vi "6240AData_execute.vi"(0 "6240AData in":refnum<class "6240AData.lvclass">, 5 "SetCurrent (A)":dbl[](array[numeric]), 7 "FileFormat":string, 9 "Output status":bool[](array[boolean]), 10 "ExecutionIndex":i32, 11 "error in (no error)":errorcluster) -> (1 "ActualVoltage (V)":dbl[](array[numeric]), 3 "ActualCurrent (A)":dbl[](array[numeric]), 4 "6240AData out":refnum<class "6240AData.lvclass">, 6 "appended array":timestamp[](array[timestamp]), 12 "SetCurrentArray":dbl[][](array[numeric]), 14 "ActualCurrentArray":dbl[][](array[numeric]), 15 "error out":errorcluster)   [LabVIEW 2020, in "6240AData.lvclass"]
uses:
  6240AData.lvclass
  6240AData.lvclass/6240AData.ctl
  istr.lib/ADCMT 6240/Public/Configure/Configure Output Mode (DC).vi
  istr.lib/ADCMT 6240/Public/Action-Status/Output (Suspend).vi
  istr.lib/ADCMT 6240/Public/Action-Status/Output (Operate).vi
  istr.lib/ADCMT 6240/ADCMT 6240.lvlib
panel:
  out "appended array 2":dbl[](array[numeric])
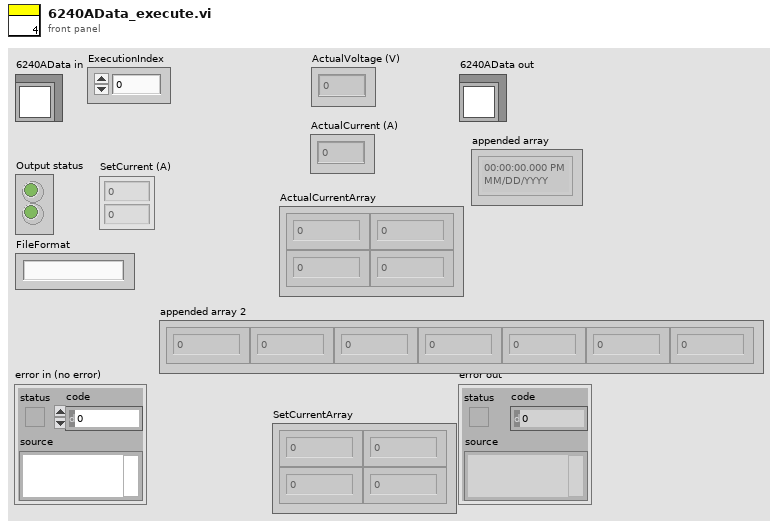
[diagram p1: front panel]
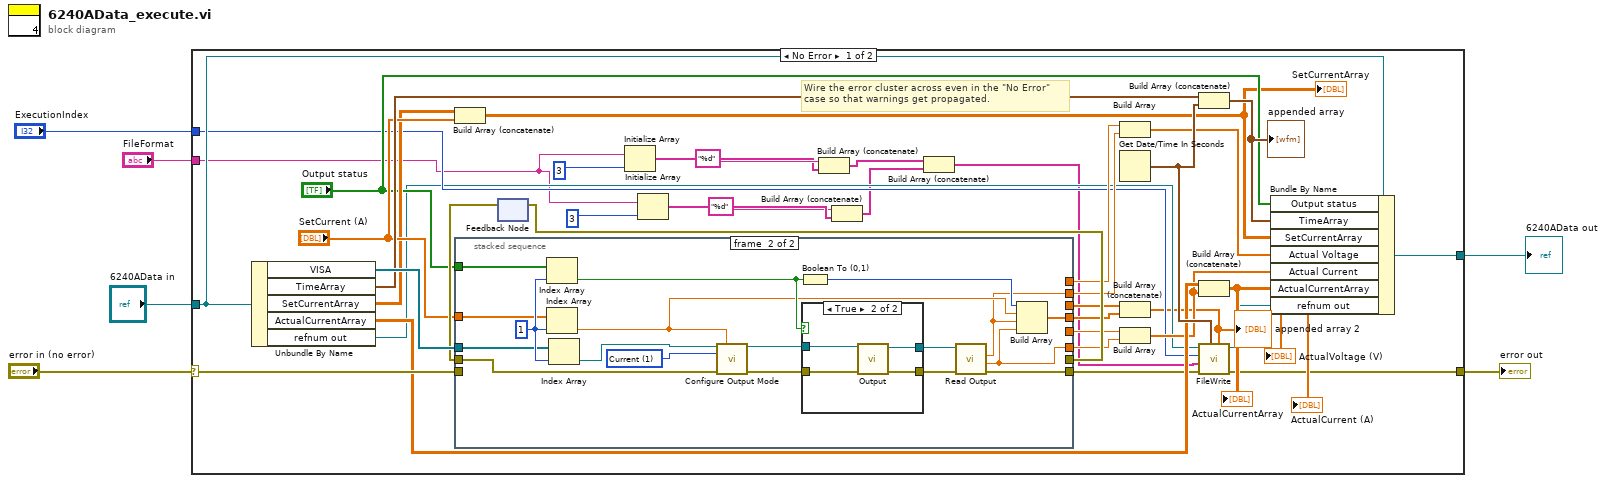
[diagram p0: block diagram]
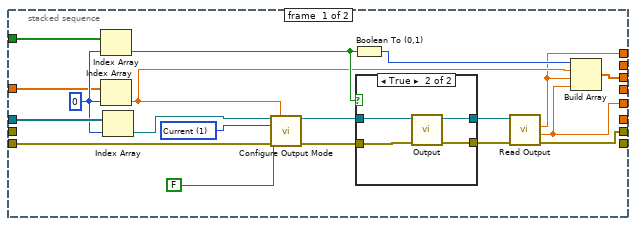
[diagram p2: hidden frame]
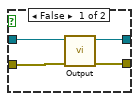
[diagram p3: hidden frame]
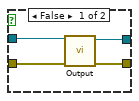
[diagram p4: hidden frame]
diagram:
  n1 = case shown="No Error" "error in (no error)" {
    selector: "error in (no error)" -> [w42 w99]
    tunnel: [w38 w100] -> w4
    tunnel: "6240AData in" -> [w41 w100]
    tunnel: [w18 w99] -> w3
    tunnel: "ExecutionIndex" -> [w24 _]
    tunnel: "FileFormat" -> [w11 _]
    frame No Error {
      # "Wire the error cluster across even in the \"No Error\"\ncase so that warnings get propagated."
      n2 = Unbundle By Name(w41) -> ("VISA"=w45:refnum<visa-resource-name>[], "TimeArray"=w40:timestamp[], "SetCurrentArray"=w31:dbl[][], "ActualCurrentArray"=w30:dbl[][], "refnum out"=w23:refnum<file>)
      n3 = Build Array (concatenate)(w31, "SetCurrent (A)") -> (w16:dbl[][])
      "SetCurrentArray" <- w16
      n4 = feedback #1() -> (w43:errorcluster)  [unwired: 1 in]
      n5 = stacked-sequence {
        tunnel: w45 -> [w61 w83]
        tunnel: "Output status" -> [w59 w82]
        tunnel: [w55 _] -> w44
        tunnel: w43 -> [_ w85]
        tunnel: w42 -> [w54 _]
        tunnel: [_ w80] -> w26
        tunnel: "SetCurrent (A)" -> [w53 w79]
        tunnel: [w49 _] -> w36
        tunnel: [_ w75] -> w35
        tunnel: [w48 _] -> w34
        tunnel: [_ w74] -> w33
        tunnel: [w47 _] -> w21
        tunnel: [_ w73] -> w20
        frame #0 {
          w58 = 0 ("index")
          w64 = 1 items=["Voltage", "Current"] ("Source Function  (0: Voltage)")
          n6 = Index Array(array=w59, index=w58) -> (element=w52:bool)
          n7 = Index Array(array=w53, index=w58) -> (element=w50:dbl)
          n8 = Index Array(array=w61, index=w58) -> (element=w60:refnum<visa-resource-name>)
          n9 = call-poly "Configure Output Mode.vi"("VISA resource name"=w60, "Output Value (0.0)"=w50, "Source Function  (0: Voltage)"=w64, "Enable Manual Range (F: Disable)"=FALSE, "error in (no error)"=w54) -> ("VISA resource name out"=w63:refnum<visa-resource-name>, "error out"=w62:errorcluster)  [unwired: 9 in]
          n10 = Boolean To (0,1)(Boolean=w52) -> (0, 1=w51:i16)
          n11 = case shown="True" w52 {
            tunnel: w63 -> [w68 w72]
            tunnel: w62 -> [w67 w71]
            tunnel: [w66 w70] -> w56
            tunnel: [w65 w69] -> w57
            frame False {
              n12 = call-poly "Output.vi"("error in (no error)"=w67, "VISA resource name"=w68) -> ("error out"=w66:errorcluster, "VISA resource name out"=w65:refnum<visa-resource-name>)  [unwired: 8 in]
            }
            frame True {
              n13 = call-poly "Output.vi"("error in (no error)"=w71, "VISA resource name"=w72) -> ("error out"=w70:errorcluster, "VISA resource name out"=w69:refnum<visa-resource-name>)  [unwired: 8 in]
            }
          }
          n14 = call "Read Output.vi"("error in (no error)"=w56, "VISA resource name"=w57) -> ("error out"=w55:errorcluster, "Actual Current Level (A)"=w48:dbl, "Actual Voltage Level (V)"=w49:dbl)  [unwired: 6 in, 1 out]
          n15 = Build Array(w51, w50, w49, w48) -> (w47:dbl[])
        }
        frame #1 {
          w84 = 1 ("index")
          w90 = 1 items=["Voltage", "Current"] ("Source Function  (0: Voltage)")
          n16 = Index Array(array=w82, index=w84) -> (element=w78:bool)
          n17 = Index Array(array=w79, index=w84) -> (element=w76:dbl)
          n18 = Index Array(array=w83, index=w84) -> (element=w81:refnum<visa-resource-name>)
          n19 = call-poly "Configure Output Mode.vi"("VISA resource name"=w81, "Output Value (0.0)"=w76, "Source Function  (0: Voltage)"=w90, "error in (no error)"=w85) -> ("VISA resource name out"=w89:refnum<visa-resource-name>, "error out"=w88:errorcluster)  [unwired: 10 in]
          n20 = Boolean To (0,1)(Boolean=w78) -> (0, 1=w77:i16)
          n21 = case shown="True" w78 {
            tunnel: w89 -> [w94 w98]
            tunnel: w88 -> [w93 w97]
            tunnel: [w92 w96] -> w86
            tunnel: [w91 w95] -> w87
            frame False {
              n22 = call-poly "Output.vi"("error in (no error)"=w93, "VISA resource name"=w94) -> ("error out"=w92:errorcluster, "VISA resource name out"=w91:refnum<visa-resource-name>)  [unwired: 8 in]
            }
            frame True {
              n23 = call-poly "Output.vi"("error in (no error)"=w97, "VISA resource name"=w98) -> ("error out"=w96:errorcluster, "VISA resource name out"=w95:refnum<visa-resource-name>)  [unwired: 8 in]
            }
          }
          n24 = call "Read Output.vi"("error in (no error)"=w86, "VISA resource name"=w87) -> ("error out"=w80:errorcluster, "Actual Current Level (A)"=w74:dbl, "Actual Voltage Level (V)"=w75:dbl)  [unwired: 6 in, 1 out]
          n25 = Build Array(w77, w76, w75, w74) -> (w73:dbl[])
        }
      }
      n26 = feedback-in #1(w44) -> ()
      n27 = Initialize Array(w11, 3 ("dimension size")) -> (w14:string[])
      n28 = Initialize Array(w11, 3 ("dimension size")) -> (w13:string[])
      n29 = Build Array (concatenate)("%d", w14) -> (w10:string[])
      n30 = Build Array (concatenate)("%d", w13) -> (w9:string[])
      n31 = Build Array (concatenate)(w10, w9) -> (w8:string[])
      n32 = Build Array(w36, w35) -> (w17:dbl[])
      "ActualVoltage (V)" <- w17
      n33 = Get Date/Time In Seconds() -> (seconds since 1Jan1904=w39:timestamp)
      n34 = Build Array (concatenate)(w21, w20) -> (w19:dbl[])
      "appended array 2" <- w19
      n35 = Build Array(w34, w33) -> (w29:dbl[])
      "ActualCurrent (A)" <- w29
      n36 = Build Array (concatenate)(w40, w39) -> (w37:timestamp[])
      "appended array" <- w37
      n37 = Build Array (concatenate)(w30, w29) -> (w28:dbl[][])
      "ActualCurrentArray" <- w28
      n38 = call "FileWrite.vi"("DataArray"=w19, "Time Stamp"=w39, "Error In"=w26, "FileFormat"=w8, "Index"=w24, "refnum in"=w23) -> ("Error Out"=w18:errorcluster, "Byte Stream File Refnum"=w27:refnum<file>)  [unwired: 4 in]
      n39 = Bundle By Name(cluster=w41, "Output status"="Output status", "TimeArray"=w37, "SetCurrentArray"=w16, "Actual Voltage"=w17, "Actual Current"=w29, "ActualCurrentArray"=w28, "refnum out"=w27) -> (w38:refnum<class "6240AData.lvclass">)
    }
    frame Error {
    }
  }
  "error out" <- w3
  "6240AData out" <- w4
